vi "Read Taus.vi"() -> ()   [LabVIEW 2012]
uses:
  <vilib>/Utility/file.llb/Write To Spreadsheet File (DBL).vi
panel:
  in  "Write":bool
  out "Reading":bool
  in  "clear":bool
  in  "Channel":T1(ring)
  out "plot":cluster{timestamp[], dbl[]}(graph)
  in  "plot":bool
  in  "analyze":bool
  in  "stop":bool
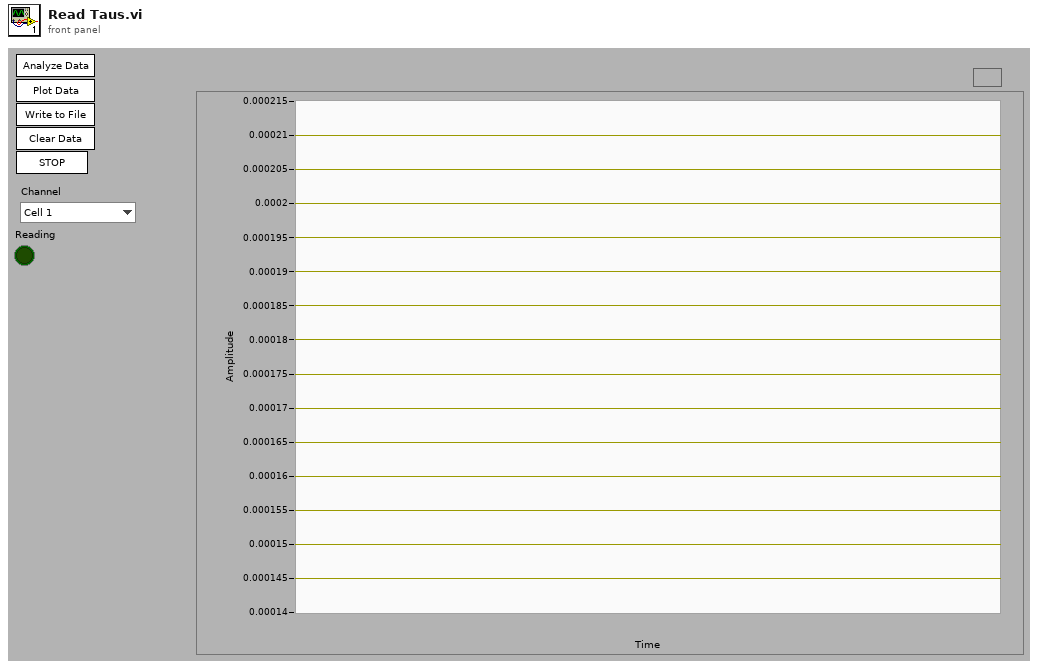
[diagram p1: front panel]
types:
  T1 = enum16{"Cell 1", "Cell 2", "Cell 3", "Cell 4", "Cell 5", "Cell 6", "Cell 7", "Cell 8"}
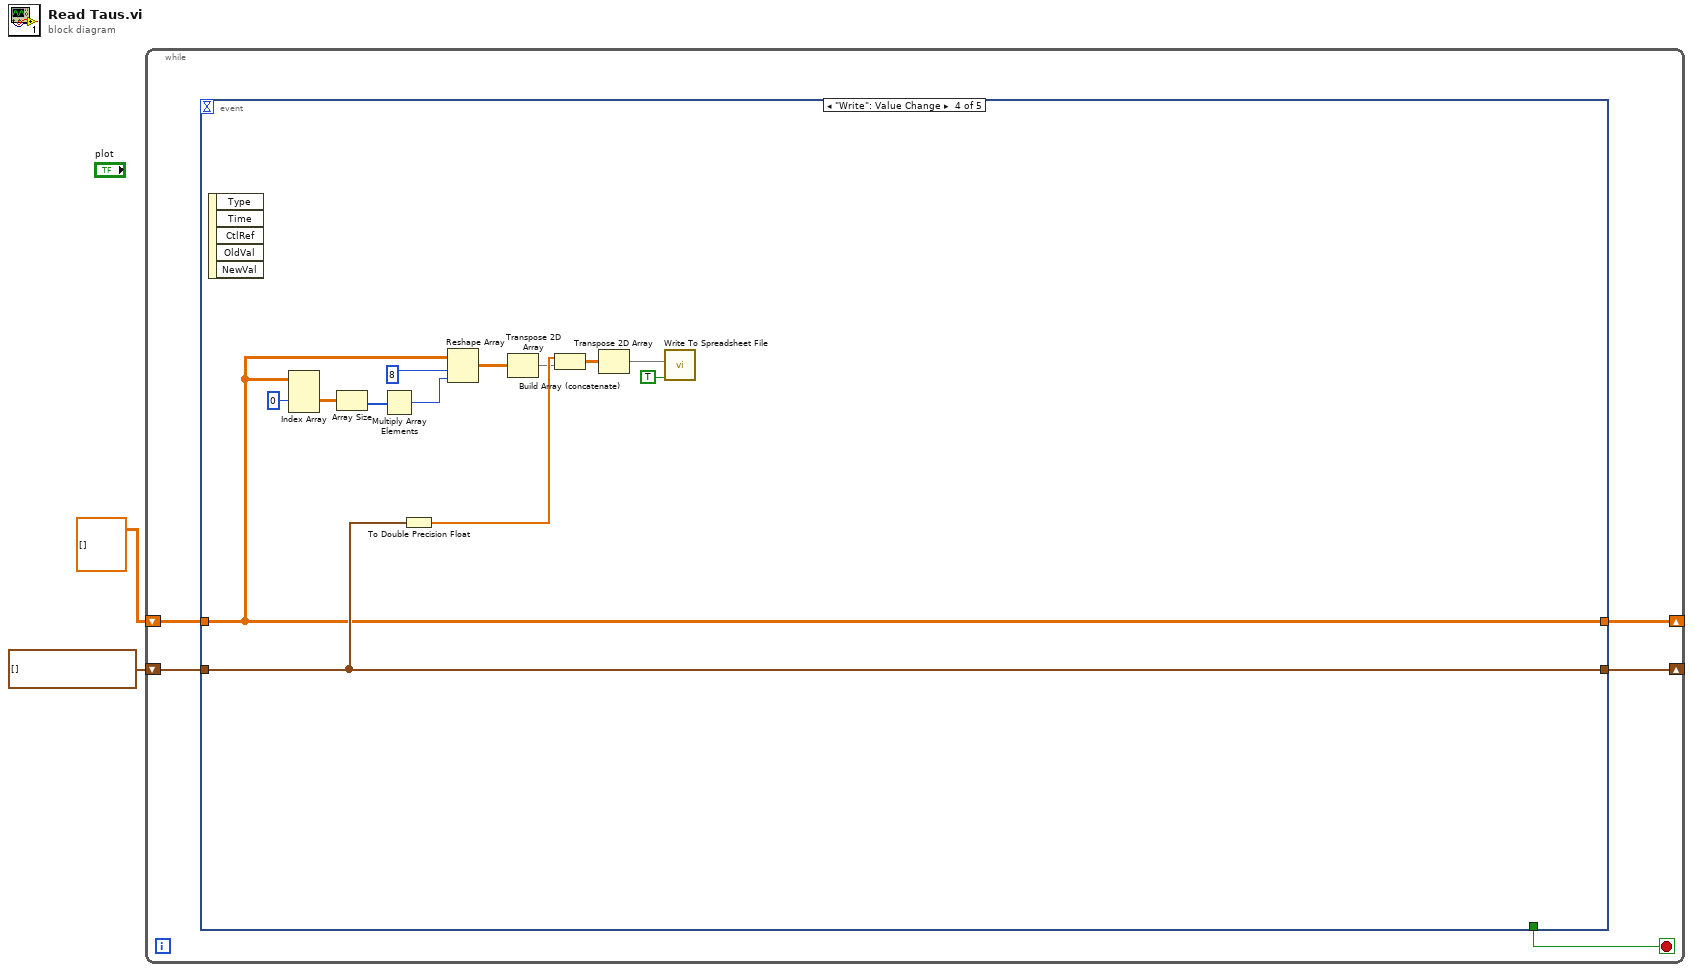
[diagram p0: block diagram]
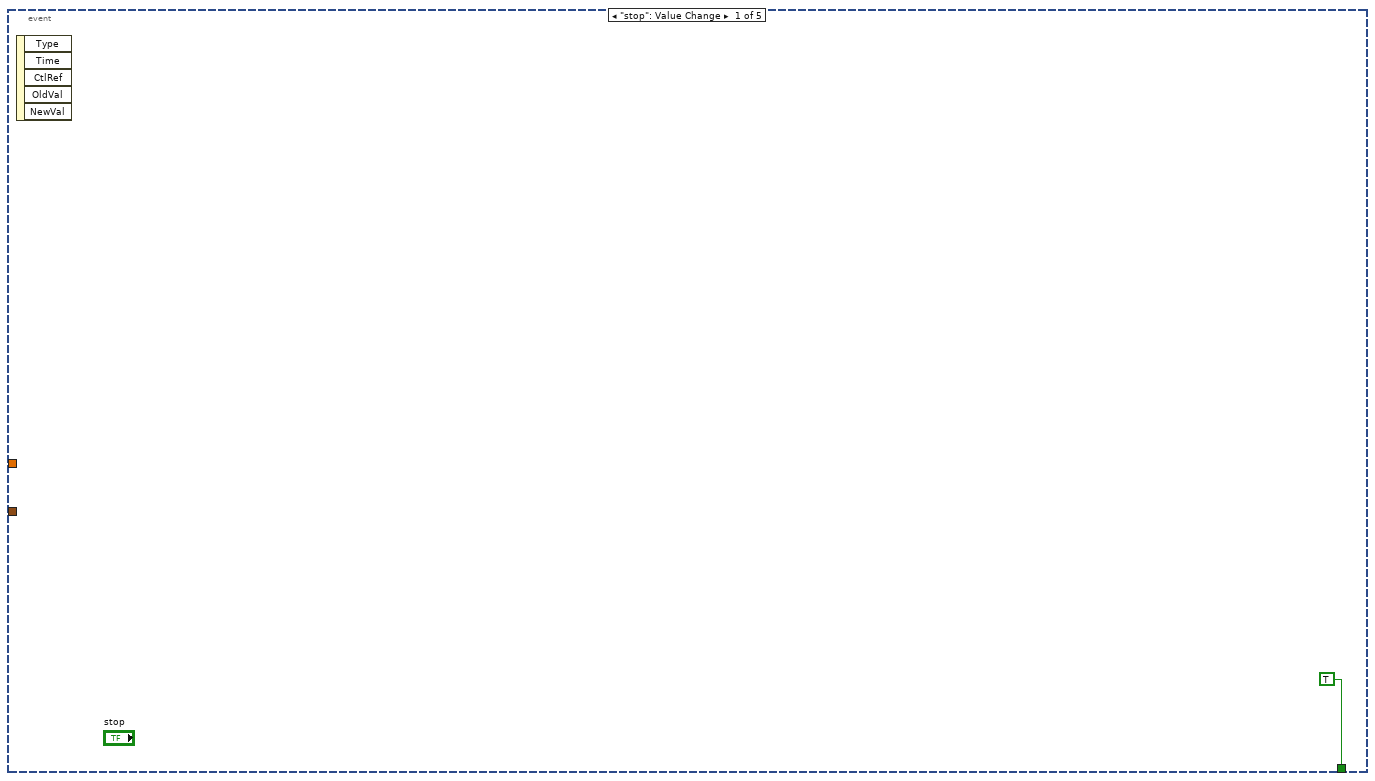
[diagram p2: hidden frame]
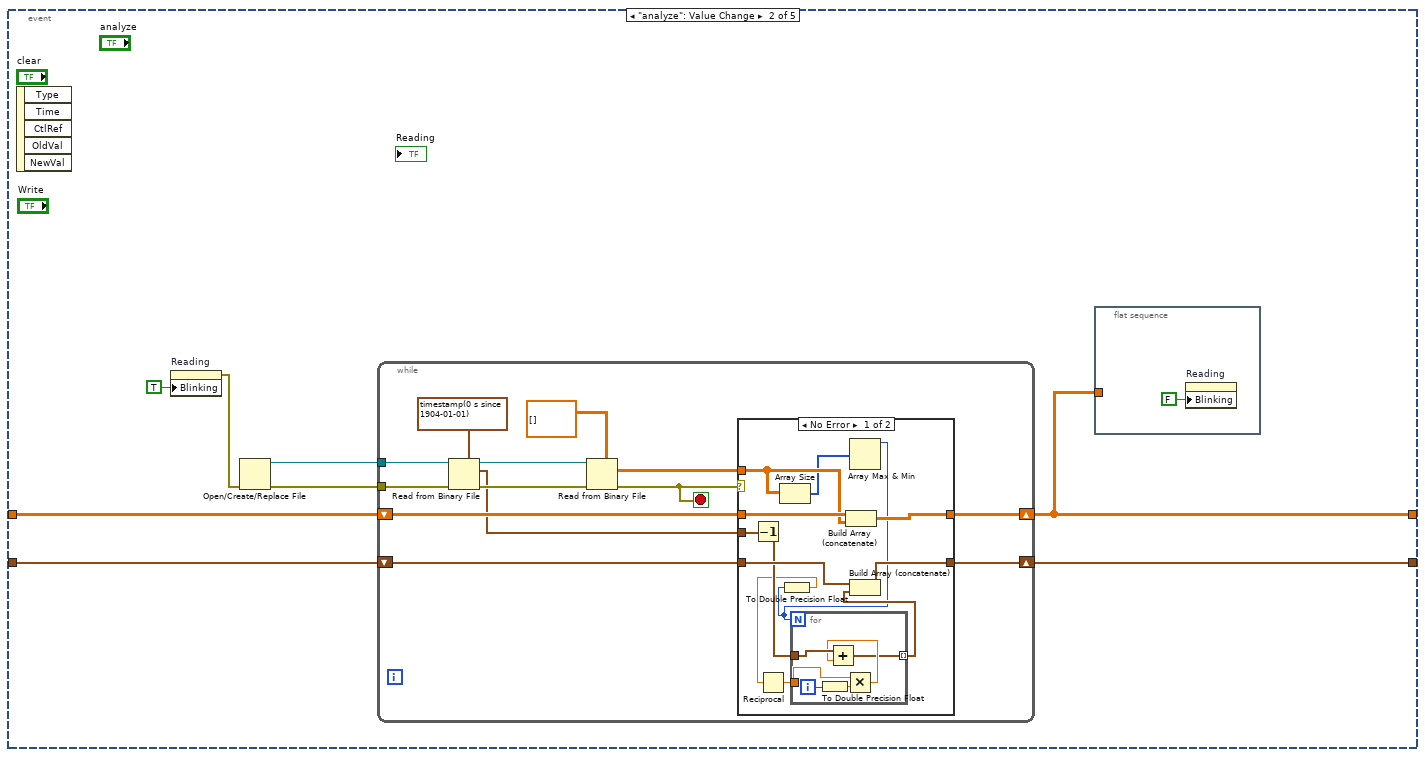
[diagram p3: hidden frame]
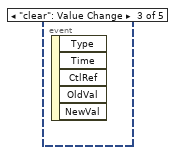
[diagram p5: hidden frame]
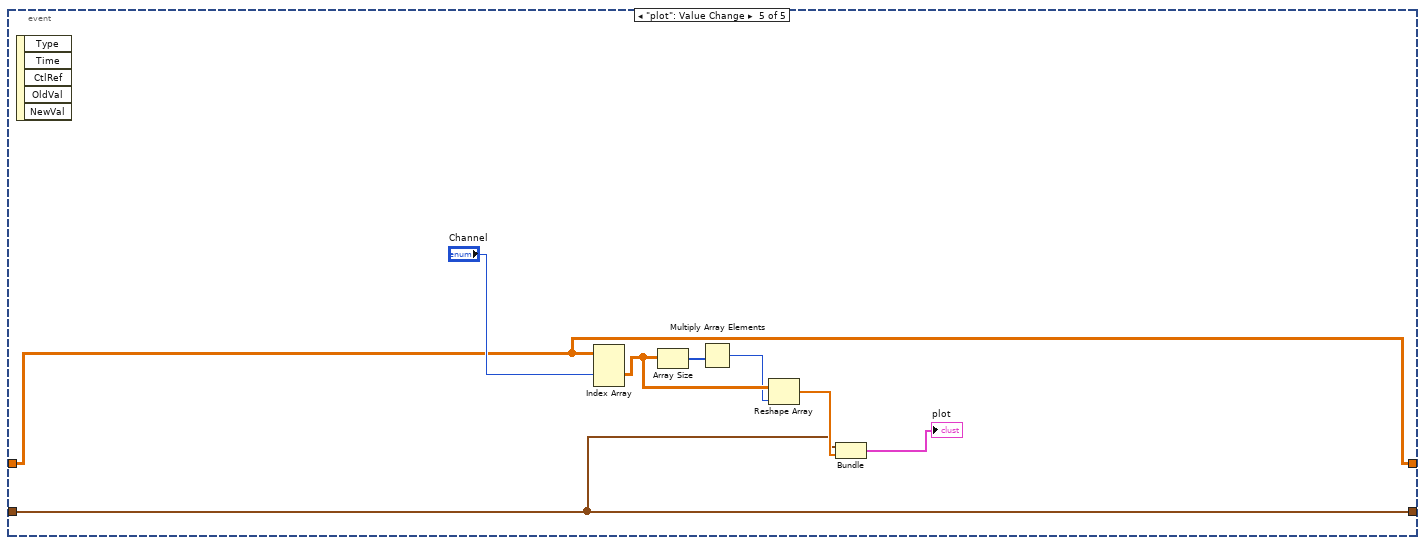
[diagram p6: hidden frame]
diagram:
  n1 = while {
    shift-right: [w5] -> _
    shift-left: dbl[][][] [] -> [w6]
    shift-right: [w4] -> _
    shift-left: timestamp[] [] -> [w3]
    stop <- w7 stop-if-true
    n2 = event shown="[3] \"Write\": Value Change" {
      selector: _ -> [_ _ _ _ _]
      dyn-events: _ -> [_ _ _ _ _]
      timeout: _ -> [_ _ _ _ _]
      tunnel: [TRUE _ _ _ _] -> w7
      tunnel: w6 -> [_ w13 _ w61 w65]
      tunnel: [_ w9 _ w61 w65] -> w5
      tunnel: [_ w14 _ w63 w66] -> w4
      tunnel: w3 -> [_ w12 _ w63 w66]
      event "stop": Value Change {
        n3 = event-data() -> ()  [unwired: 1 in, 5 out]
      }
      event "analyze": Value Change {
        n4 = event-data() -> ()  [unwired: 1 in, 5 out]
        n5 = property on="Reading" class="Bool (strict)"("Blinking"=TRUE) -> (error out=w10:errorcluster)  [unwired: 2 in, 1 out]
        n6 = Open/Create/Replace File(error in=w10) -> (refnum out=w16:refnum<file>, error out=w15:errorcluster)  [unwired: 5 in, 1 out]
        n7 = while {
          tunnel: w16 -> [w30]
          tunnel: w15 -> [w29]
          shift-right: [w21] -> w9
          shift-left: w13 -> [w23]
          shift-right: [w19] -> w14
          shift-left: w12 -> [w20]
          stop <- w24 stop-if-true
          n8 = Read from Binary File(5:timestamp(0 s since 1904-01-01), 8:w29, 11:w30) -> (0:w26:errorcluster, 2:w18:timestamp, 3:w27:refnum<file>)  [unwired: 3 in, 1 out]
          n9 = Read from Binary File(5:dbl[][] [], 8:w26, 11:w27) -> (0:w24:errorcluster, 2:w22:dbl[][])  [unwired: 3 in, 2 out]
          n10 = case shown="No Error" w24 {
            tunnel: w23 -> [w42 w50]
            tunnel: w22 -> [w37 _]
            tunnel: [w41 w50] -> w21
            tunnel: w20 -> [w40 w49]
            tunnel: [w39 w49] -> w19
            tunnel: w18 -> [w38 _]
            frame No Error {
              n11 = Decrement(x=w38) -> (x-1=w35:timestamp)
              n12 = Array Size(array=w37) -> (size(s)=w36:i32[])
              n13 = Build Array (concatenate)(w42, w37) -> (w41:dbl[][][])
              n14 = Array Max & Min(array=w36) -> (max value=w32:i32)  [unwired: 3 out]
              n15 = To Double Precision Float(number=w32) -> (double precision float=w31:dbl)
              n16 = Reciprocal(x=w31) -> (1/x=w34:dbl)
              n17 = for {
                N: w32 -> [_]
                tunnel: w35 -> [w48]
                tunnel: w34 -> [w47]
                tunnel: [w43] -> w33 mode=indexing
                i -> [w46]
                n18 = To Double Precision Float(number=w46) -> (double precision float=w45:dbl)
                n19 = Multiply(x=w47, y=w45) -> (x*y=w44:dbl)
                n20 = Add(x=w48, y=w44) -> (x+y=w43:timestamp)
              }
              n21 = Build Array (concatenate)(w40, w33) -> (w39:timestamp[])
            }
            frame Error {
            }
          }
        }
        n22 = flat-sequence {
          tunnel: w9 -> [_]
          frame #0 {
            n23 = property on="Reading" class="Bool (strict)"("Blinking"=FALSE) -> ()  [unwired: 2 in, 2 out]
          }
        }
      }
      event "clear": Value Change {
        n24 = event-data() -> ()  [unwired: 1 in, 5 out]
      }
      event "Write": Value Change {
        n25 = event-data() -> ()  [unwired: 1 in, 5 out]
        n26 = Index Array(array=w61, index (dim 1)=0 ("disabled index (row)")) -> (element=w59:dbl[][])  [unwired: 2 in]
        n27 = Array Size(array=w59) -> (size(s)=w58:i32[])
        n28 = Multiply Array Elements(1:w58) -> (0:w57:i32)
        n29 = To Double Precision Float(number=w63) -> (double precision float=w55:dbl[])
        n30 = Reshape Array(w61, 8 ("dimension size"), w57) -> (w56:dbl[][])
        n31 = Transpose 2D Array(2D array=w56) -> (transposed array=w54:dbl[][])
        n32 = Build Array (concatenate)(w55, w54) -> (w53:dbl[][])
        n33 = Transpose 2D Array(2D array=w53) -> (transposed array=w52:dbl[][])
        n34 = call-poly <vilib>:"Write To Spreadsheet File.vi"("append to file? (new file:F)"=TRUE, "2D data"=w52) -> ()  [unwired: 6 in, 1 out]
      }
      event "plot": Value Change {
        n35 = event-data() -> ()  [unwired: 1 in, 5 out]
        n36 = Index Array(array=w65, index (dim 1)="Channel") -> (element=w69:dbl[][])  [unwired: 2 in]
        n37 = Array Size(array=w69) -> (size(s)=w70:i32[])
        n38 = Multiply Array Elements(1:w70) -> (0:w64:i32)
        n39 = Reshape Array(w69, w64) -> (w68:dbl[])
        n40 = Bundle(w66, w68) -> (→"plot":cluster{timestamp[], dbl[]})  [unwired: 1 in]
      }
    }
  }
